vi "Util_ConvertArrayOfPathsToArrayOfStringPaths.vi"(1 "PathsArray":path[](array[path])) -> (0 "ArrayOfStringPaths":string[](array[string]))   [LabVIEW 2023]
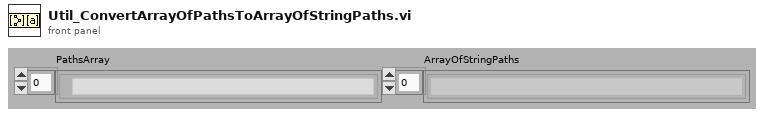
[diagram p1: front panel]
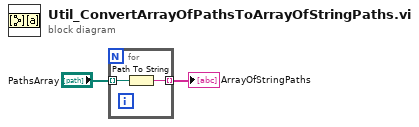
[diagram p0: block diagram]
diagram:
  n1 = for {
    tunnel: "PathsArray" -> [w4] mode=indexing
    tunnel: [w3] -> w1 mode=indexing
    n2 = Path To String(path=w4) -> (string=w3:string)
  }
  "ArrayOfStringPaths" <- w1
